vi "CRYSet Drop Data.vi"(11 "Graph Type In":string) -> (3 "Graph Type Out":string)   [LabVIEW 2013]
uses:
  CRYWindow/DataView/Control/CRYDrag Graph.ctl
  CRYWindow/DataView/SubVI/CRYData View Global.vi
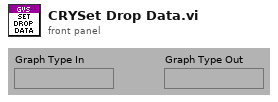
[diagram p1: front panel]
types:
  T1 = typedef "CRYDrag Graph.ctl" = cluster{"GraphType":string, "GraphData":variant}
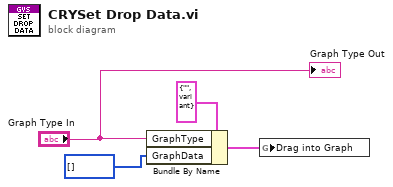
[diagram p0: block diagram]
diagram:
  n1 = Bundle By Name(cluster=T1 {"GraphType"="", "GraphData"=variant} ("Drag Graph Cluster"), "GraphType"="Graph Type In", "GraphData"=i32[] [] ("Drag Rows")) -> (w2:T1)
  n2 = global write "CRYData View Global.vi" "Drag into Graph"(w2) -> ()
  "Graph Type Out" <- "Graph Type In"
